vi "CAN read.vi"(6 "error in (no error)":errorcluster, 9 "CANopen in":refnum<class "CANopen.lvclass">) -> (0 "error out":errorcluster, 1 "Data":u8[](array[numeric]), 2 "COB id":i32, 3 "CANopen out":refnum<class "CANopen.lvclass">, 4 "No data?":bool)   [LabVIEW 2017, in "canopen.lvlib" / "CANopen.lvclass"]
doc: "Returns the oldest COB present in the reception queue."
uses:
  CANopen.lvclass
  CANopen.lvclass/CANopen.ctl
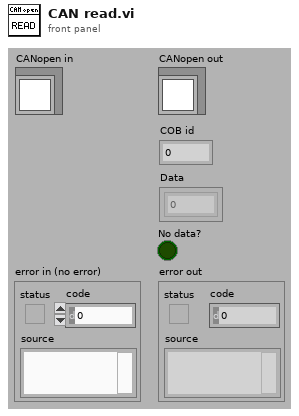
[diagram p1: front panel]
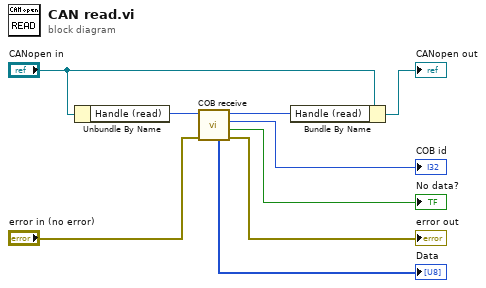
[diagram p0: block diagram]
diagram:
  n1 = Unbundle By Name("CANopen in") -> ("Handle (read)"=w7:i32)
  n2 = call "COB receive.vi"("error in (no error)"="error in (no error)", "Handle in"=w7) -> ("error out"=→"error out":errorcluster, "No data?"=→"No data?":bool, "COB id"=→"COB id":i32, "Handle out"=w6:i32, "Data"=→"Data":u8[])  [unwired: 3 out]
  n3 = Bundle By Name(cluster="CANopen in", "Handle (read)"=w6) -> (→"CANopen out":refnum<class "CANopen.lvclass">)
